vi "ARDUINO PID AJUSTE GANANCIAS.vi"() -> ()   [LabVIEW 2024]
uses:
  <vilib>/Instr/_visa.llb/VISA Configure Serial Port (Instr).vi
panel:
  in  "kd":dbl
  in  "kp":dbl
  in  "ki":dbl
  in  "stop":bool
  in  "th_des":u16(knob) scale=0.0..360.0
  in  "VISA resource name":refnum<visa-resource-name>
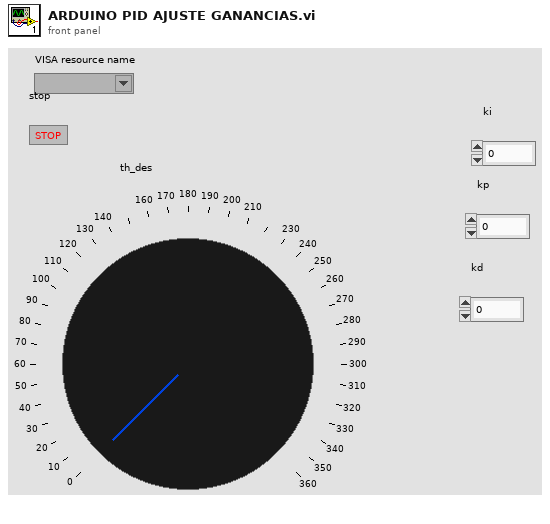
[diagram p1: front panel]
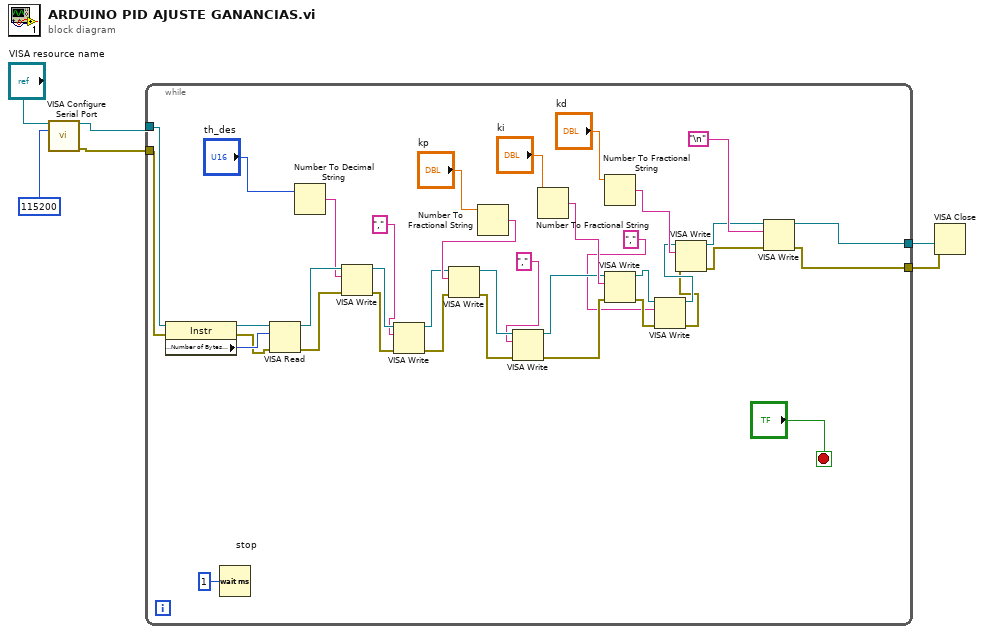
[diagram p0: block diagram]
diagram:
  n1 = call-poly "VISA Configure Serial Port"("VISA resource name"="VISA resource name", "baud rate (9600)"=u32 115200) -> ("VISA resource name out"=w6:refnum<visa-resource-name>, "error out"=w5:errorcluster)  [unwired: 12 in]
  n2 = while {
    tunnel: w6 -> [w40]
    tunnel: w5 -> [w39]
    tunnel: [w26] -> w2
    tunnel: [w25] -> w1
    stop <- "stop" stop-if-true
    n3 = property class="Instr"(reference=w40, error in=w39) -> (reference out=w43:refnum<visa-resource-name>, error out=w41:errorcluster, "Serial Settings:Number of Bytes at Serial Port"=w42:u32)
    n4 = Wait (ms)(milliseconds to wait=u32 1) -> ()  [unwired: 1 out]
    n5 = VISA Read(VISA resource name=w43, byte count=w42, error in (no error)=w41) -> (VISA resource name out=w38:refnum<visa-resource-name>, error out=w37:errorcluster)  [unwired: 2 out]
    n6 = Number To Decimal String(number="th_des") -> (decimal integer string=w36:string)  [unwired: 1 in]
    n7 = VISA Write(VISA resource name=w38, write buffer=w36, error in (no error)=w37) -> (VISA resource name out=w11:refnum<visa-resource-name>, error out=w10:errorcluster)  [unwired: 1 out]
    n8 = VISA Write(VISA resource name=w11, write buffer=",", error in (no error)=w10) -> (VISA resource name out=w12:refnum<visa-resource-name>, error out=w13:errorcluster)  [unwired: 1 out]
    n9 = Number To Fractional String(number="kp") -> (F-format string=w31:string)  [unwired: 3 in]
    n10 = VISA Write(VISA resource name=w12, write buffer=w31, error in (no error)=w13) -> (VISA resource name out=w15:refnum<visa-resource-name>, error out=w14:errorcluster)  [unwired: 1 out]
    n11 = VISA Write(VISA resource name=w15, write buffer=",", error in (no error)=w14) -> (VISA resource name out=w16:refnum<visa-resource-name>, error out=w17:errorcluster)  [unwired: 1 out]
    n12 = Number To Fractional String(number="ki") -> (F-format string=w29:string)  [unwired: 3 in]
    n13 = Number To Fractional String(number="kd") -> (F-format string=w27:string)  [unwired: 3 in]
    n14 = VISA Write(VISA resource name=w16, write buffer=w29, error in (no error)=w17) -> (VISA resource name out=w19:refnum<visa-resource-name>, error out=w18:errorcluster)  [unwired: 1 out]
    n15 = VISA Write(VISA resource name=w19, write buffer=",", error in (no error)=w18) -> (VISA resource name out=w21:refnum<visa-resource-name>, error out=w20:errorcluster)  [unwired: 1 out]
    n16 = VISA Write(VISA resource name=w21, write buffer=w27, error in (no error)=w20) -> (VISA resource name out=w22:refnum<visa-resource-name>, error out=w23:errorcluster)  [unwired: 1 out]
    n17 = VISA Write(VISA resource name=w22, write buffer="\n", error in (no error)=w23) -> (VISA resource name out=w26:refnum<visa-resource-name>, error out=w25:errorcluster)  [unwired: 1 out]
  }
  n18 = VISA Close(VISA resource name=w2, error in (no error)=w1) -> ()  [unwired: 1 out]
